vi "SpecVals.vi"(5 "df":dbl, 6 "2nd freq":dbl, 7 "window":i32=2, 8 "Tone Burst":dbl[](array[numeric]), 9 "Power Spectrum":dbl[](array[numeric])) -> (0 "x < 0?":bool, 1 "diff":dbl, 2 "2nd f db":dbl, 3 "40 Mhz db":dbl, 4 "MSE":dbl format="%0.2f")   [LabVIEW 2022 SP3]
uses:
  <vilib>/Analysis/baseanly.llb/Mean (DBL).vi
  <vilib>/Analysis/NI_AALPro.lvlib
  <vilib>/Analysis/NI_AALBase.lvlib
panel:
  in  "Quad MSE":dbl=0.1
  in  "Fun MSE thresh":dbl=0.1
  out "Polynomial Fit Coefficients 2":dbl[](array[numeric]) format="%0.2f"
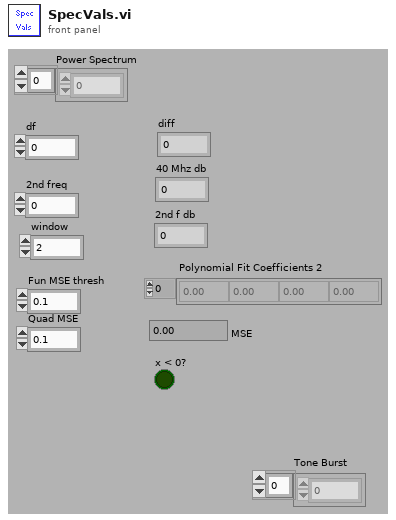
[diagram p1: front panel]
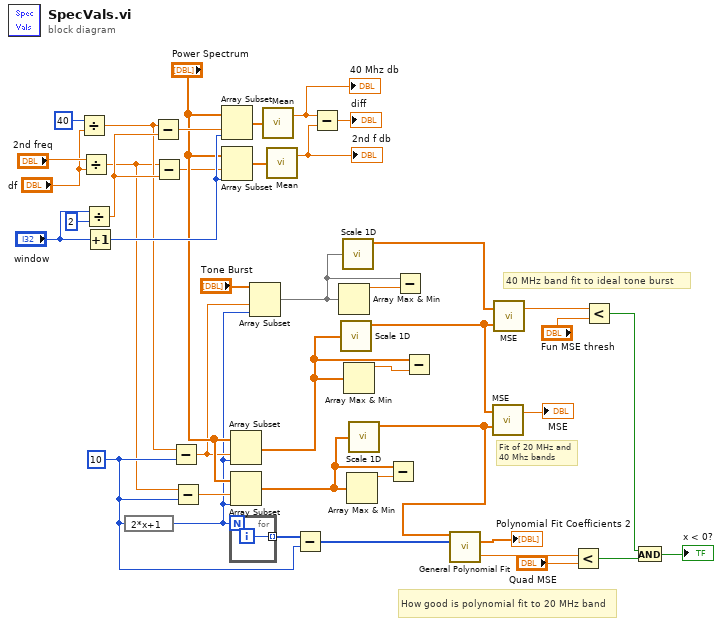
[diagram p0: block diagram]
diagram:
  w21 = 10
  # "How good is polynomial fit to 20 MHz band"
  # "Fit of 20 MHz and 40 Mhz bands"
  # "40 MHz band fit to ideal tone burst"
  n1 = Divide(x=40, y="df") -> (x/y=w2:dbl)
  n2 = Divide(x="2nd freq", y="df") -> (x/y=w1:dbl)
  n3 = Divide(x="window", y=2) -> (x/y=w32:dbl)
  n4 = Increment(x="window") -> (x+1=w33:i32)
  n5 = expression code="2*x+1"(w21) -> (w17:i32)
  n6 = Subtract(x=w2, y=w32) -> (x-y=w30:dbl)
  n7 = Subtract(x=w1, y=w32) -> (x-y=w25:dbl)
  n8 = Subtract(x=w2, y=w21) -> (x-y=w18:dbl)
  n9 = Subtract(x=w1, y=w21) -> (x-y=w29:dbl)
  n10 = Array Subset(array="Power Spectrum", index=w30, length=w33) -> (w40:dbl[])
  n11 = Array Subset(array="Power Spectrum", index=w25, length=w33) -> (w31:dbl[])
  n12 = for {
    N: w17 -> [_]
    tunnel: [w43] -> w27 mode=indexing
    i -> [w43]
  }
  n13 = Array Subset(array="Power Spectrum", index=w18, length=w17) -> (w11:dbl[])
  n14 = Array Subset(array="Power Spectrum", index=w29, length=w17) -> (w8:dbl[])
  n15 = Array Subset(array="Tone Burst", index=w18, length=w17) -> (w12:dbl[])
  n16 = call-poly <vilib>:"Mean.vi"("X"=w40) -> ("mean"=w35:dbl)  [unwired: 1 out]
  "40 Mhz db" <- w35
  n17 = call-poly <vilib>:"Mean.vi"("X"=w31) -> ("mean"=w34:dbl)  [unwired: 1 out]
  "2nd f db" <- w34
  n18 = Subtract(x=w27, y=w21) -> (x-y=w26:i32[])
  n19 = Subtract(x=w35, y=w34) -> (x-y=→"diff":dbl)
  n20 = Array Max & Min(array=w12) -> (max value=w16:dbl)  [unwired: 3 out]
  n21 = call <vilib>:"Scale 1D.vi"("X"=w11) -> ("Y=(X-offset)/scale"=w6:dbl[])  [unwired: 3 out]
  n22 = call <vilib>:"Scale 1D.vi"("X"=w12) -> ("Y=(X-offset)/scale"=w10:dbl[])  [unwired: 3 out]
  n23 = Array Max & Min(array=w11) -> (max value=w23:dbl)  [unwired: 3 out]
  n24 = Array Max & Min(array=w8) -> (max value=w22:dbl)  [unwired: 3 out]
  n25 = call <vilib>:"Scale 1D.vi"("X"=w8) -> ("Y=(X-offset)/scale"=w4:dbl[])  [unwired: 3 out]
  n26 = Subtract(x=w8, y=w22) -> ()  [unwired: 1 out]
  n27 = Subtract(x=w12, y=w16) -> ()  [unwired: 1 out]
  n28 = Subtract(x=w11, y=w23) -> ()  [unwired: 1 out]
  n29 = call <vilib>:"General Polynomial Fit.vi"("Y"=w4, "X"=w26) -> ("Polynomial Coefficients"=→"Polynomial Fit Coefficients 2":dbl[], "residue"=w5:dbl)  [unwired: 10 in, 2 out]
  n30 = call <vilib>:"MSE.vi"("X Values"=w4, "Y Values"=w6) -> ("mse"=→"MSE":dbl)  [unwired: 1 out]
  n31 = call <vilib>:"MSE.vi"("X Values"=w6, "Y Values"=w10) -> ("mse"=w9:dbl)  [unwired: 1 out]
  n32 = Less?(x=w5, y="Quad MSE") -> (x < y?=w14:bool)
  n33 = Less?(x=w9, y="Fun MSE thresh") -> (x < y?=w15:bool)
  n34 = And(x=w15, y=w14) -> (x .and. y?=→"x < 0?":bool)
